vi "Seconds to Time String.vi"(2 "error in":errorcluster, 3 "Seconds in":i32) -> (0 "error out":errorcluster, 1 "String":string)   [LabVIEW 2015]
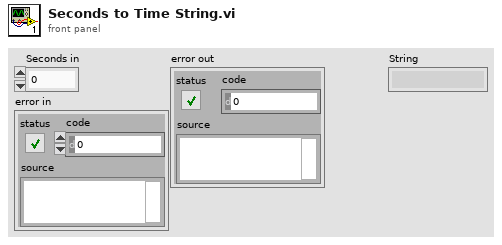
[diagram p1: front panel]
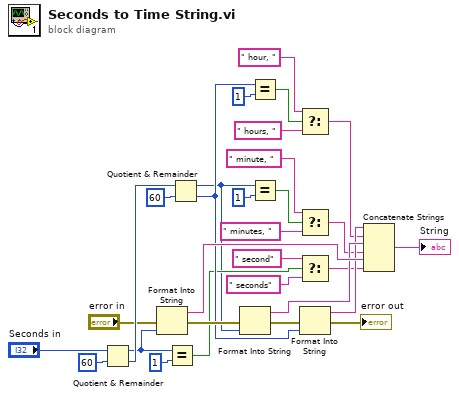
[diagram p0: block diagram]
diagram:
  n1 = Quotient & Remainder(x="Seconds in", y=60) -> (x-y*floor(x/y)=w5:i32, floor(x/y)=w28:i32)
  n2 = Format Into String(error in="error in", w5) -> (resulting string=w26:string, error out=w24:errorcluster)  [unwired: 2 in]
  n3 = Equal?(x=w5, y=1) -> (x = y?=w10:bool)
  n4 = Quotient & Remainder(x=w28, y=60) -> (x-y*floor(x/y)=w4:i32, floor(x/y)=w13:i32)
  n5 = Format Into String(error in=w24, w4) -> (resulting string=w21:string, error out=w23:errorcluster)  [unwired: 2 in]
  n6 = Equal?(x=w13, y=1) -> (x = y?=w18:bool)
  n7 = Equal?(x=w4, y=1) -> (x = y?=w12:bool)
  n8 = Select(t=" hour, " ("string"), s=w18, f=" hours, " ("string")) -> (s? t:f=w14:string)
  n9 = Select(t=" minute, " ("string"), s=w12, f=" minutes, " ("string")) -> (s? t:f=w1:string)
  n10 = Select(t=" second" ("string"), s=w10, f=" seconds" ("string")) -> (s? t:f=w6:string)
  n11 = Format Into String(error in=w23, w13) -> (resulting string=w20:string, error out=→"error out":errorcluster)  [unwired: 2 in]
  n12 = Concatenate Strings(w20, w14, w21, w1, w26, w6) -> (→"String":string)
